vi "I2C Next State Controller.vi"(7 "Execute?":bool, 8 "I2C Configuration":T1, 9 "SCL_IN":bool, 10 "SDA_IN":bool, 11 "Status":T4) -> (1 "SCL_OUT":bool, 3 "Control":T2)   [LabVIEW 2017]
uses:
  I2C Status Signals.ctl
  I2C States.ctl
  I2C Control Signals.ctl
  I2C Configuration.ctl
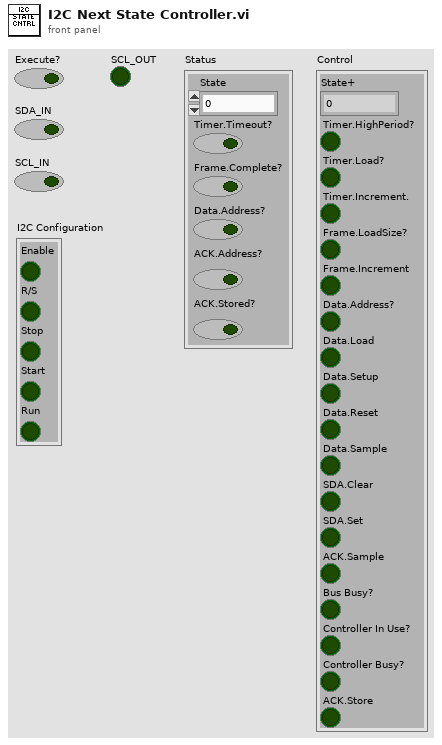
[diagram p1: front panel]
types:
  T1 = typedef "I2C Configuration.ctl" = cluster{"Enable":bool, "R/S":bool, "Stop":bool, "Start":bool, "Run":bool}
  T2 = typedef "I2C Control Signals.ctl" = cluster{"State+":T3, "Timer.HighPeriod?":bool, "Timer.Load?":bool, "Timer.Increment.":bool, "Frame.LoadSize?":bool, "Frame.Increment":bool, "Data.Address?":bool, "Data.Load":bool, "Data.Setup":bool, "Data.Reset":bool, "Data.Sample":bool, "SDA.Clear":bool, "SDA.Set":bool, "ACK.Sample":bool, "Bus Busy?":bool, "Controller In Use?":bool, "Controller Busy?":bool, "ACK.Store":bool}
  T3 = typedef "I2C States.ctl" = fxp<+,5,5>
  T4 = typedef "I2C Status Signals.ctl" = cluster{"State":T3, "Timer.Timeout?":bool, "Frame.Complete?":bool, "Data.Address?":bool, "ACK.Address?":bool, "ACK.Stored?":bool}
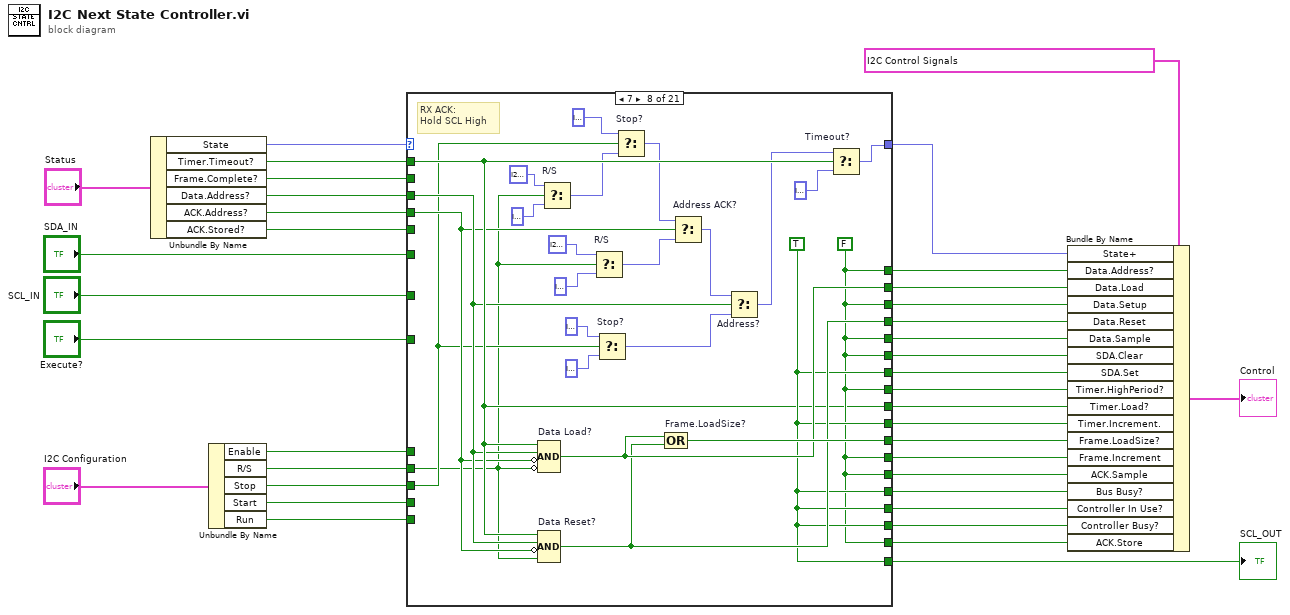
[diagram p0: block diagram]
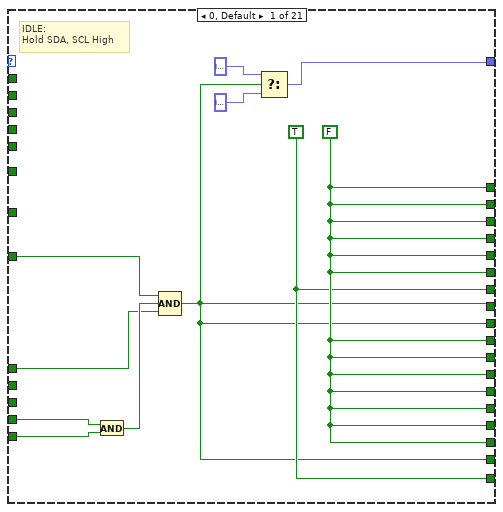
[diagram p2: hidden frame]
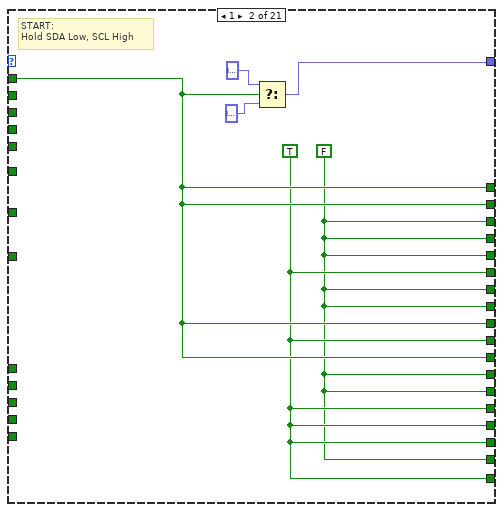
[diagram p3: hidden frame]
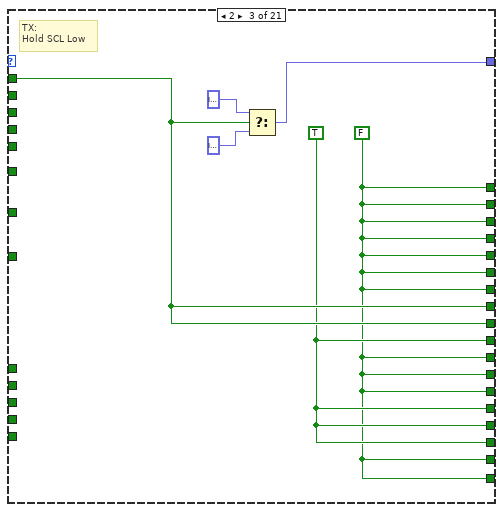
[diagram p4: hidden frame]
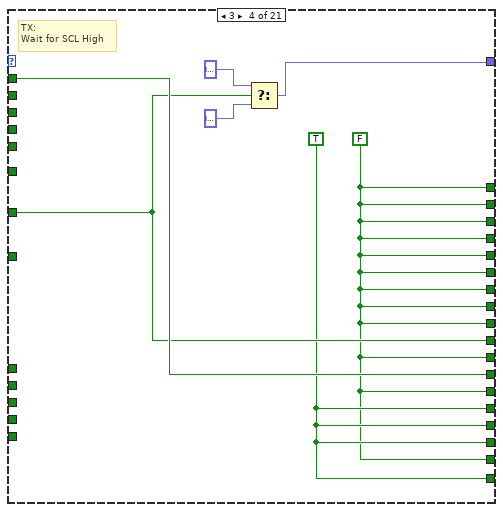
[diagram p5: hidden frame]
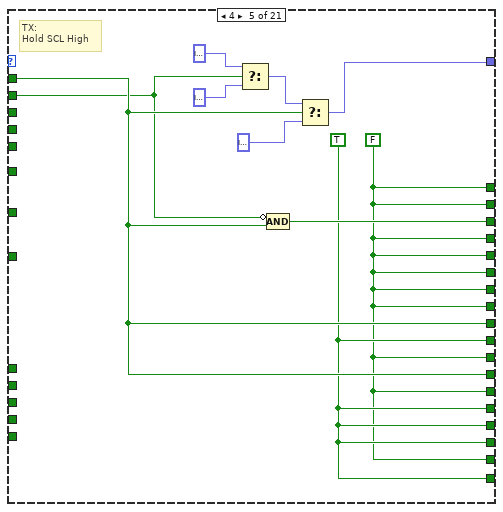
[diagram p6: hidden frame]
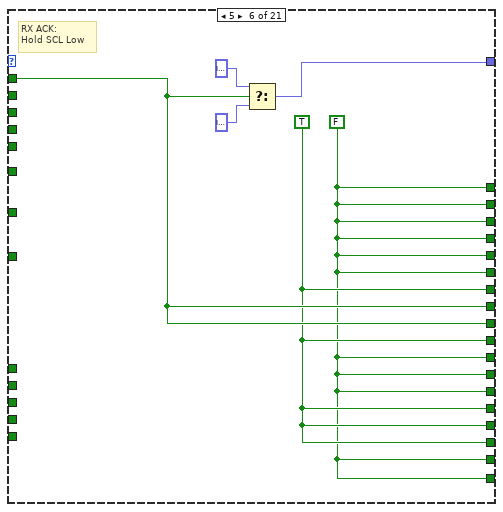
[diagram p7: hidden frame]
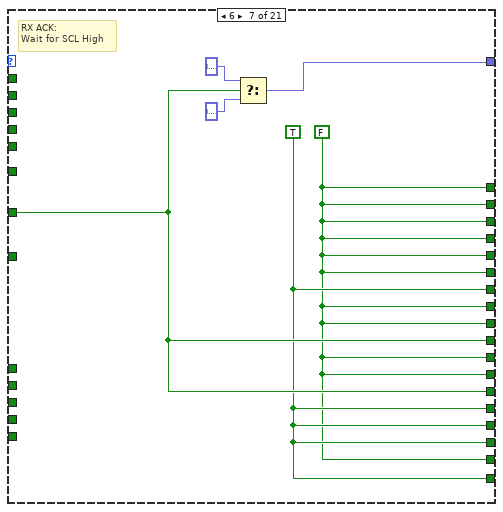
[diagram p8: hidden frame]
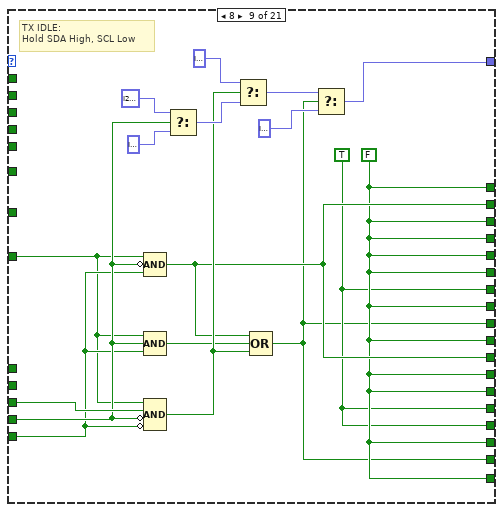
[diagram p9: hidden frame]
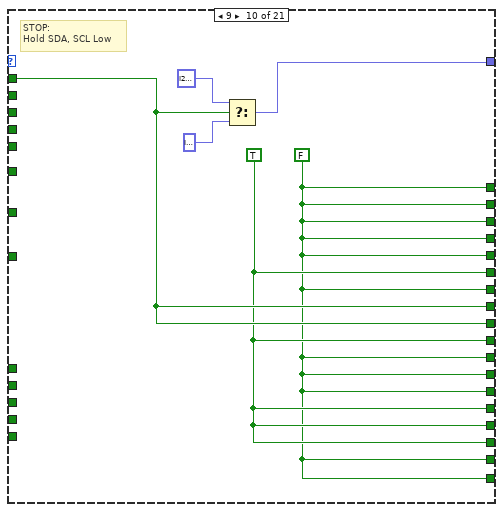
[diagram p10: hidden frame]
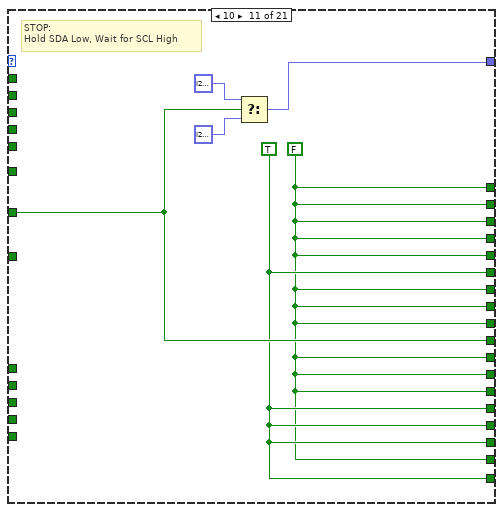
[diagram p11: hidden frame]
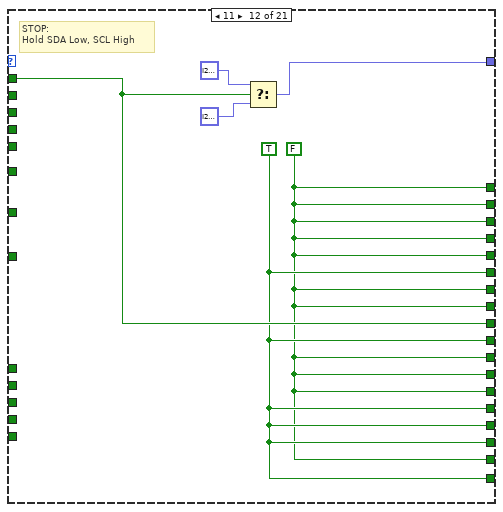
[diagram p12: hidden frame]
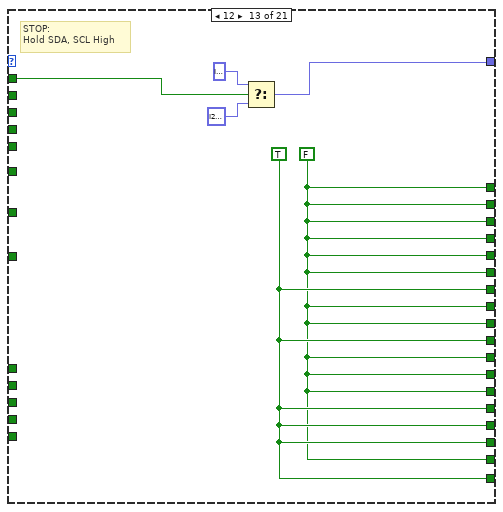
[diagram p13: hidden frame]
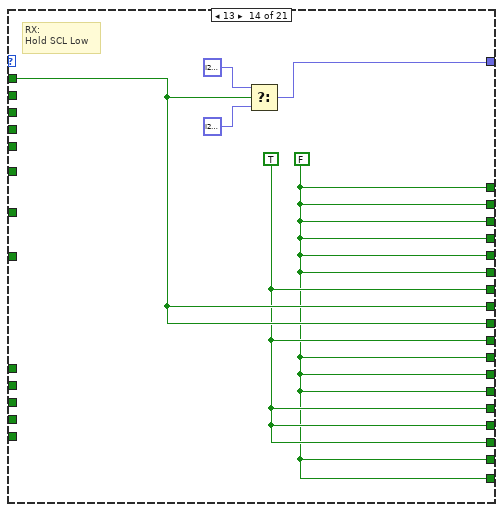
[diagram p14: hidden frame]
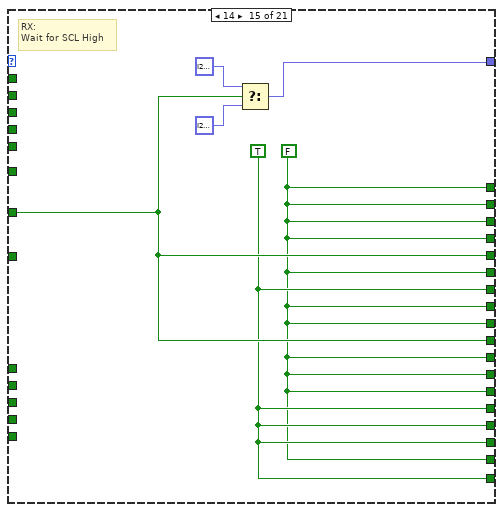
[diagram p15: hidden frame]
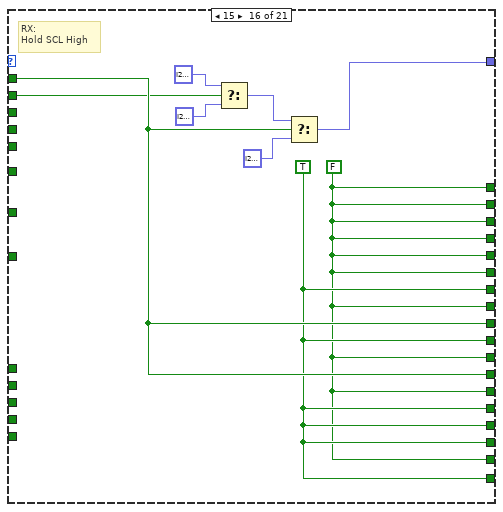
[diagram p16: hidden frame]
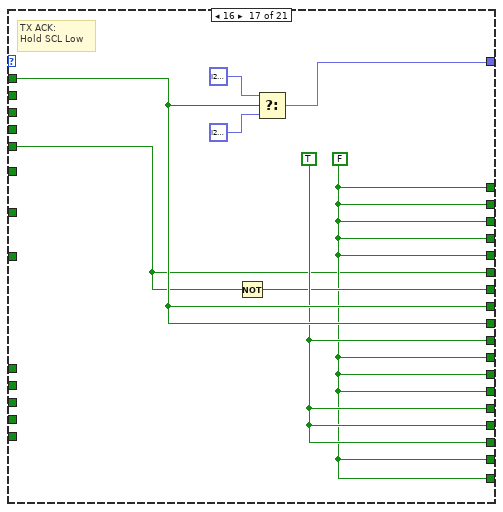
[diagram p17: hidden frame]
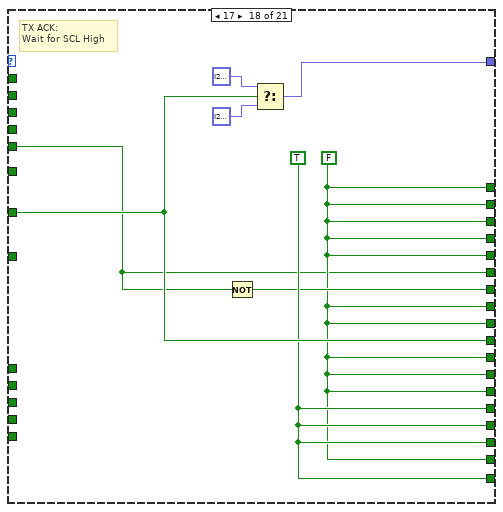
[diagram p18: hidden frame]
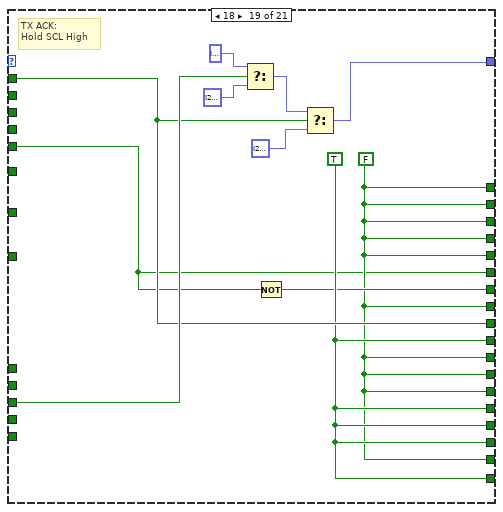
[diagram p19: hidden frame]
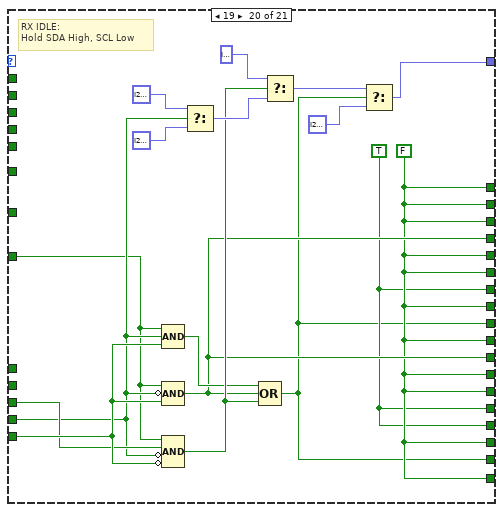
[diagram p20: hidden frame]
diagram:
  n1 = Unbundle By Name("Status") -> ("State"=w34:T3, "Timer.Timeout?"=w33:bool, "Frame.Complete?"=w32:bool, "Data.Address?"=w24:bool, "ACK.Address?"=w3:bool, "ACK.Stored?"=w1:bool)
  n2 = Unbundle By Name("I2C Configuration") -> ("Enable"=w4:bool, "R/S"=w22:bool, "Stop"=w19:bool, "Start"=w20:bool, "Run"=w21:bool)
  n3 = case shown="7" w34 {
    tunnel: "Execute?" -> [w43 _ _ _ _ _ _ _ w118 _ _ _ _ _ _ _ _ _ _ w205 _]
    tunnel: [w41 w51 w55 w61 w68 w78 w84 w113 w123 w132 w138 w144 w150 w156 w162 w168 w178 w186 w194 w210 w221] -> w12
    tunnel: [w46 w52 w58 w67 w77 w80 w87 w114 w130 w135 w141 w146 w153 w159 w165 w175 w183 w191 w202 w214 w224] -> w8
    tunnel: w33 -> [_ w51 w57 w65 w71 w83 _ w107 _ w134 _ w147 w152 w158 _ w174 w182 _ w197 _ w222]
    tunnel: w32 -> [_ _ _ _ w70 _ _ _ _ _ _ _ _ _ _ w170 _ _ _ _ _]
    tunnel: [w41 w50 w56 w63 w69 w79 w86 w110 w117 w133 w140 w145 w151 w157 w164 w169 w180 w189 w196 w209 w223] -> w9
    tunnel: [w41 w49 w55 w65 w71 w78 w84 w109 w117 w132 w138 w144 w150 w156 w162 w174 w178 w186 w194 w209 w221] -> w13
    tunnel: [w38 w49 w57 w61 w68 w83 w84 w109 w117 w134 w138 w144 w150 w158 w162 w168 w182 w186 w194 w209 w222] -> w10
    tunnel: [w38 w51 w57 w61 w71 w83 w84 w107 w115 w134 w138 w147 w150 w158 w162 w174 w182 w186 w197 w204 w222] -> w11
    tunnel: [w39 w50 w55 w62 w69 w78 w85 w110 w117 w132 w139 w145 w151 w156 w163 w169 w178 w188 w196 w209 w223] -> w36
    tunnel: "SCL_IN" -> [_ _ _ w63 _ _ w86 _ _ _ w140 _ _ _ w164 _ _ w189 _ _ _]
    tunnel: "SDA_IN" -> [_ _ _ _ _ _ _ _ _ _ _ _ _ _ _ _ _ _ _ _ _]
    tunnel: [w41 w51 w55 w61 w68 w78 w84 w109 w117 w132 w138 w144 w150 w156 w162 w168 w178 w186 w194 w209 w221] -> w27
    tunnel: [w41 w51 w55 w61 w68 w78 w84 w112 w123 w132 w138 w144 w150 w156 w162 w168 w178 w186 w194 w209 w221] -> w26
    tunnel: [w41 w49 w55 w61 w72 w78 w84 w109 w117 w132 w138 w144 w150 w156 w162 w168 w178 w186 w194 w209 w221] -> w25
    tunnel: [w41 w50 w55 w61 w68 w78 w84 w109 w117 w133 w139 w145 w150 w156 w162 w168 w177 w185 w193 w209 w221] -> w17
    tunnel: [w39 w49 w55 w61 w68 w79 w85 w110 w116 w132 w138 w144 w151 w157 w163 w169 w179 w187 w195 w208 w223] -> w18
    tunnel: [w41 w49 w55 w61 w68 w78 w86 w109 w117 w132 w138 w144 w150 w156 w162 w168 w178 w186 w194 w209 w221] -> w14
    tunnel: w24 -> [_ _ _ _ _ _ _ w106 _ _ _ _ _ _ _ _ _ _ _ _ _]
    tunnel: w22 -> [_ _ _ _ _ _ _ w95 _ _ _ _ _ _ _ _ _ _ _ _ _]
    tunnel: w19 -> [_ _ _ _ _ _ _ w96 w121 _ _ _ _ _ _ _ _ _ w198 w207 _]
    tunnel: w20 -> [w45 _ _ _ _ _ _ _ w120 _ _ _ _ _ _ _ _ _ _ w206 _]
    tunnel: w21 -> [w44 _ _ _ _ _ _ _ w119 _ _ _ _ _ _ _ _ _ _ w213 _]
    tunnel: [w41 w49 w55 w61 w68 w78 w84 w109 w117 w132 w138 w144 w150 w156 w164 w168 w178 w186 w194 w209 w221] -> w16
    tunnel: [w41 w49 w55 w61 w68 w78 w84 w111 w117 w132 w138 w144 w150 w156 w162 w168 w178 w186 w194 w210 w221] -> w15
    tunnel: [w41 w50 w56 w62 w69 w79 w85 w110 w116 w133 w139 w145 w151 w157 w163 w169 w180 w188 w196 w208 w223] -> w7
    tunnel: [w41 w50 w56 w62 w69 w79 w85 w110 w116 w133 w139 w145 w151 w157 w163 w169 w180 w188 w196 w208 w223] -> w6
    tunnel: [w41 w50 w56 w62 w69 w79 w85 w110 w117 w133 w139 w145 w151 w157 w163 w169 w180 w188 w196 w209 w223] -> w5
    tunnel: w4 -> [w40 _ _ _ _ _ _ _ _ _ _ _ _ _ _ _ _ _ _ _ _]
    tunnel: w3 -> [_ _ _ _ _ _ _ w100 _ _ _ _ _ _ _ _ _ _ _ _ _]
    tunnel: [w38 w49 w55 w61 w68 w78 w84 w109 w115 w132 w138 w144 w150 w156 w162 w168 w178 w186 w194 w204 w221] -> w2
    tunnel: w1 -> [_ _ _ _ _ _ _ _ _ _ _ _ _ _ _ _ w177 w185 w193 _ _]
    frame 0, Default {
      w39 = TRUE ("Start?")
      w41 = FALSE ("Increment")
      # "IDLE:\nHold SDA, SCL High"
      n4 = And(x=w45, y=w44) -> (x .and. y?=w42:bool)
      n5 = Compound Arithmetic op=AND(w43, w42, w40) -> (w38:bool)
      n6 = Select(t=T3 1.0 ("State+"), s=w38, f=T3 0.0 ("State+")) -> (s? t:f=w46:T3)
    }
    frame 1 {
      w50 = TRUE ("Start?")
      w49 = FALSE ("Increment")
      # "START:\nHold SDA Low, SCL High"
      n7 = Select(t=T3 2.0 ("State+"), s=w51, f=T3 1.0 ("State+")) -> (s? t:f=w52:T3)
    }
    frame 2 {
      w56 = TRUE ("Start?")
      w55 = FALSE ("Start?")
      # "TX:\nHold SCL Low"
      n8 = Select(t=T3 3.0 ("State+"), s=w57, f=T3 2.0 ("State+")) -> (s? t:f=w58:T3)
    }
    frame 3 {
      w62 = TRUE ("Start?")
      w61 = FALSE ("Start?")
      # "TX:\nWait for SCL High"
      n9 = Select(t=T3 4.0 ("State+"), s=w63, f=T3 3.0 ("State+")) -> (s? t:f=w67:T3)
    }
    frame 4 {
      w69 = TRUE ("Start?")
      w68 = FALSE ("Start?")
      # "TX:\nHold SCL High"
      n10 = Select(t=T3 5.0 ("State+"), s=w70, f=T3 2.0 ("State+")) -> (s? t:f=w73:T3)
      n11 = Compound Arithmetic op=AND(invert w70, w71) -> (w72:bool)
      n12 = Select(t=w73, s=w71, f=T3 4.0 ("State+")) -> (s? t:f=w77:T3)
    }
    frame 5 {
      w78 = FALSE ("Start?")
      w79 = TRUE ("Start?")
      # "RX ACK:\nHold SCL Low"
      n13 = Select(t=T3 6.0 ("State+"), s=w83, f=T3 5.0 ("State+")) -> (s? t:f=w80:T3)
    }
    frame 6 {
      w84 = FALSE ("Start?")
      w85 = TRUE ("Start?")
      # "RX ACK:\nWait for SCL High"
      n14 = Select(t=T3 7.0 ("State+"), s=w86, f=T3 6.0 ("State+")) -> (s? t:f=w87:T3)
    }
    frame 7 {
      w109 = FALSE ("Start?")
      w110 = TRUE ("Start?")
      # "RX ACK:\nHold SCL High"
      n15 = Compound Arithmetic op=AND "Data Load?"(w107, w106, invert w100, invert w95) -> (w112:bool)
      n16 = Compound Arithmetic op=AND "Data Reset?"(w107, w106, invert w100, w95) -> (w111:bool)
      n17 = Select "R/S"(t=T3 19.0 ("State+"), s=w95, f=T3 8.0) -> (s? t:f=w92:T3)
      n18 = Select "R/S"(t=T3 13.0 ("State+"), s=w95, f=T3 2.0) -> (s? t:f=w99:T3)
      n19 = Select "Stop?"(t=T3 9.0 ("State+"), s=w96, f=T3 8.0) -> (s? t:f=w103:T3)
      n20 = Select "Stop?"(t=T3 9.0, s=w96, f=w92) -> (s? t:f=w90:T3)
      n21 = Compound Arithmetic op=OR "Frame.LoadSize?"(w112, w111) -> (w113:bool)
      n22 = Select "Address ACK?"(t=w90, s=w100, f=w99) -> (s? t:f=w98:T3)
      n23 = Select "Address?"(t=w98, s=w106, f=w103) -> (s? t:f=w97:T3)
      n24 = Select "Timeout?"(t=w97, s=w107, f=T3 7.0 ("State+")) -> (s? t:f=w114:T3)
    }
    frame 8 {
      w116 = TRUE ("Start?")
      w117 = FALSE ("Start?")
      # "TX IDLE:\nHold SDA High, SCL Low"
      n25 = Compound Arithmetic op=AND(w118, invert w120, w119) -> (w123:bool)
      n26 = Compound Arithmetic op=AND(w118, w120, w119) -> (w122:bool)
      n27 = Compound Arithmetic op=AND(w118, w121, invert w120, invert w119) -> (w124:bool)
      n28 = Select(t=T3 20.0 ("State+"), s=w120, f=T3 2.0 ("State+")) -> (s? t:f=w125:T3)
      n29 = Select(t=T3 9.0 ("State+"), s=w124, f=w125) -> (s? t:f=w126:T3)
      n30 = Compound Arithmetic op=OR(w123, w122, w124) -> (w115:bool)
      n31 = Select(t=w126, s=w115, f=T3 8.0 ("State+")) -> (s? t:f=w130:T3)
    }
    frame 9 {
      w132 = FALSE ("Start?")
      w133 = TRUE ("Start?")
      # "STOP:\nHold SDA, SCL Low"
      n32 = Select(t=T3 10.0 ("State+"), s=w134, f=T3 9.0 ("State+")) -> (s? t:f=w135:T3)
    }
    frame 10 {
      w138 = FALSE ("Start?")
      w139 = TRUE ("Start?")
      # "STOP:\nHold SDA Low, Wait for SCL High"
      n33 = Select(t=T3 11.0 ("State+"), s=w140, f=T3 10.0 ("State+")) -> (s? t:f=w141:T3)
    }
    frame 11 {
      w144 = FALSE ("Start?")
      w145 = TRUE ("Start?")
      # "STOP:\nHold SDA Low, SCL High"
      n34 = Select(t=T3 12.0 ("State+"), s=w147, f=T3 11.0 ("State+")) -> (s? t:f=w146:T3)
    }
    frame 12 {
      w150 = FALSE ("Start?")
      w151 = TRUE ("Start?")
      # "STOP:\nHold SDA, SCL High"
      n35 = Select(t=T3 0.0 ("State+"), s=w152, f=T3 12.0 ("State+")) -> (s? t:f=w153:T3)
    }
    frame 13 {
      w156 = FALSE ("Start?")
      w157 = TRUE ("Start?")
      # "RX:\nHold SCL Low"
      n36 = Select(t=T3 14.0 ("State+"), s=w158, f=T3 13.0 ("State+")) -> (s? t:f=w159:T3)
    }
    frame 14 {
      w162 = FALSE ("Start?")
      w163 = TRUE ("Start?")
      # "RX:\nWait for SCL High"
      n37 = Select(t=T3 15.0 ("State+"), s=w164, f=T3 14.0 ("State+")) -> (s? t:f=w165:T3)
    }
    frame 15 {
      w168 = FALSE ("Start?")
      w169 = TRUE ("Start?")
      # "RX:\nHold SCL High"
      n38 = Select(t=T3 16.0 ("State+"), s=w170, f=T3 13.0 ("State+")) -> (s? t:f=w171:T3)
      n39 = Select(t=w171, s=w174, f=T3 15.0 ("State+")) -> (s? t:f=w175:T3)
    }
    frame 16 {
      w178 = FALSE ("Start?")
      w180 = TRUE ("Start?")
      # "TX ACK:\nHold SCL Low"
      n40 = Not(x=w177) -> (.not. x?=w179:bool)
      n41 = Select(t=T3 17.0 ("State+"), s=w182, f=T3 16.0 ("State+")) -> (s? t:f=w183:T3)
    }
    frame 17 {
      w186 = FALSE ("Start?")
      w188 = TRUE ("Start?")
      # "TX ACK:\nWait for SCL High"
      n42 = Not(x=w185) -> (.not. x?=w187:bool)
      n43 = Select(t=T3 18.0 ("State+"), s=w189, f=T3 17.0 ("State+")) -> (s? t:f=w191:T3)
    }
    frame 18 {
      w194 = FALSE ("Start?")
      w196 = TRUE ("Start?")
      # "TX ACK:\nHold SCL High"
      n44 = Select(t=T3 9.0 ("State+"), s=w198, f=T3 19.0 ("State+")) -> (s? t:f=w199:T3)
      n45 = Not(x=w193) -> (.not. x?=w195:bool)
      n46 = Select(t=w199, s=w197, f=T3 18.0 ("State+")) -> (s? t:f=w202:T3)
    }
    frame 19 {
      w209 = FALSE ("Start?")
      w208 = TRUE ("Start?")
      # "RX IDLE:\nHold SDA High, SCL Low"
      n47 = Compound Arithmetic op=AND(w205, w206, w213) -> (w211:bool)
      n48 = Compound Arithmetic op=AND(w205, invert w206, w213) -> (w210:bool)
      n49 = Compound Arithmetic op=AND(w205, w207, invert w206, invert w213) -> (w212:bool)
      n50 = Select(t=T3 20.0 ("State+"), s=w206, f=T3 13.0 ("State+")) -> (s? t:f=w215:T3)
      n51 = Compound Arithmetic op=OR(w211, w210, w212) -> (w204:bool)
      n52 = Select(t=T3 9.0 ("State+"), s=w212, f=w215) -> (s? t:f=w216:T3)
      n53 = Select(t=w216, s=w204, f=T3 19.0 ("State+")) -> (s? t:f=w214:T3)
    }
    frame 20 {
      w223 = TRUE ("Start?")
      w221 = FALSE ("Increment")
      # "REPEATED START:\nHold SCL, SDA High"
      n54 = Select(t=T3 1.0 ("State+"), s=w222, f=T3 20.0 ("State+")) -> (s? t:f=w224:T3)
    }
  }
  "SCL_OUT" <- w36
  n55 = Bundle By Name(cluster=T2 {"State+"=0.0, "Timer.HighPeriod?"=FALSE, "Timer.Load?"=FALSE, "Timer.Increment."=FALSE, "Frame.LoadSize?"=FALSE, "Frame.Increment"=FALSE, "Data.Address?"=FALSE, "Data.Load"=FALSE, "Data.Setup"=FALSE, "Data.Reset"=FALSE, "Data.Sample"=FALSE, "SDA.Clear"=FALSE, "SDA.Set"=FALSE, "ACK.Sample"=FALSE, "Bus Busy?"=FALSE, "Controller In Use?"=FALSE, "Controller Busy?"=FALSE, "ACK.Store"=FALSE} ("Control"), "State+"=w8, "Data.Address?"=w27, "Data.Load"=w26, "Data.Setup"=w25, "Data.Reset"=w15, "Data.Sample"=w16, "SDA.Clear"=w17, "SDA.Set"=w18, "Timer.HighPeriod?"=w10, "Timer.Load?"=w11, "Timer.Increment."=w9, "Frame.LoadSize?"=w12, "Frame.Increment"=w13, "ACK.Sample"=w14, "Bus Busy?"=w7, "Controller In Use?"=w6, "Controller Busy?"=w5, "ACK.Store"=w2) -> (→"Control":T2)
